vi "Run Type Dialog.vi"() -> (2 "Cancelled?":bool, 3 "Run Type":T1)   [LabVIEW 2019]
uses:
  Run Type.ctl
panel:
  in  "Acquire Live":bool
  in  "Acquire Simulated":bool
  in  "Process Existing":bool
  # "This option will start a new data acquisition run, and will gather data from a pair of connected Arduino sensors."
  # "This option will load data from a stored datafile, and allow adjustments of data selection."
  # "This option will start a new data acquisition run, and will gather random fake data. It should be used for testing only."
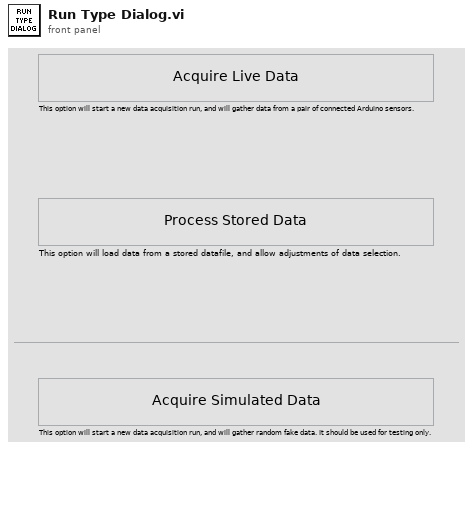
[diagram p1: front panel]
types:
  T1 = typedef "Run Type.ctl" = enum16{"Acquire - Live", "Acquire - Simulated", "Process"}
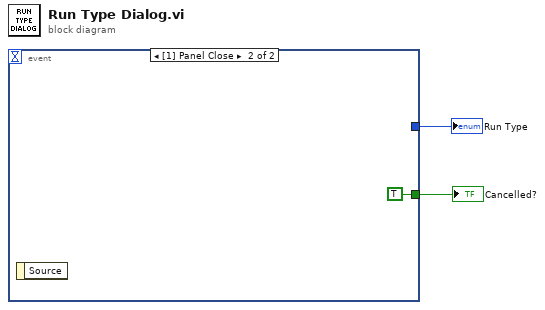
[diagram p0: block diagram]
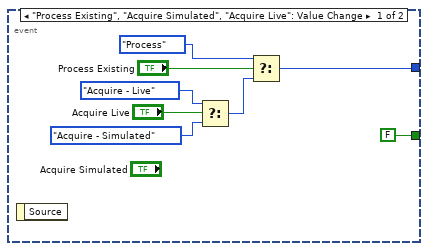
[diagram p2: hidden frame]
diagram:
  n1 = event shown="[1] Panel Close" {
    selector: _ -> [_ _]
    dyn-events: _ -> [_ _]
    timeout: _ -> [_ _]
    tunnel: [w4 _] -> w2
    tunnel: [FALSE TRUE] -> w1
    event "Process Existing", "Acquire Simulated", "Acquire Live": Value Change {
      n2 = event-data() -> ()  [unwired: 1 in, 1 out]
      n3 = Select(t=Run_Type."Acquire - Live" ("Run Type"), s="Acquire Live", f=Run_Type."Acquire - Simulated" ("Run Type")) -> (s? t:f=w6:T1)
      n4 = Select(t=Run_Type."Process" ("Run Type"), s="Process Existing", f=w6) -> (s? t:f=w4:T1)
    }
    event Panel Close {
      n5 = event-data() -> ()  [unwired: 1 in, 1 out]
    }
  }
  "Run Type" <- w2
  "Cancelled?" <- w1
